vi "test_term2.vi"   [LabVIEW 2010]
uses:
  socket_type.ctl
  zmq_context.lvclass
  zmq_socket.lvclass
  zeromq.lvlib
types:
  T1 = typedef "zeromq.lvlib/socket_type.ctl" = enum8{"ZMQ_PAIR", "ZMQ_PUB", "ZMQ_SUB", "ZMQ_REQ", "ZMQ_REP", "ZMQ_DEALER", "ZMQ_ROUTER", "ZMQ_PULL", "ZMQ_PUSH", "ZMQ_XPUB", "ZMQ_XSUB"}
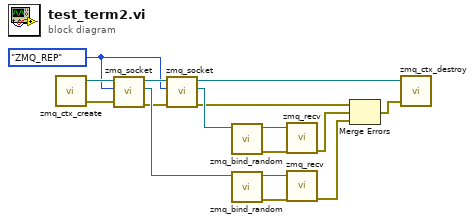
[diagram p0: block diagram]
diagram:
  w1 = socket_type."ZMQ_REP" ("socket type")
  n1 = call "zmq_ctx_create.vi"() -> ("error out"=w8:errorcluster, "context out"=w16:refnum<class "zmq_context.lvclass">)  [unwired: 4 in]
  n2 = call "zmq_socket.vi"("error in"=w8, "socket type"=w1, "context in"=w16) -> ("error out"=w7:errorcluster, "socket out"=w14:refnum<class "zmq_socket.lvclass">, "context out"=w15:refnum<class "zmq_context.lvclass">)  [unwired: 2 in]
  n3 = call "zmq_socket.vi"("error in"=w7, "socket type"=w1, "context in"=w15) -> ("error out"=w6:errorcluster, "socket out"=w13:refnum<class "zmq_socket.lvclass">, "context out"=w2:refnum<class "zmq_context.lvclass">)  [unwired: 2 in]
  n4 = call "zmq_bind_random.vi"("socket in"=w13) -> ("error out"=w12:errorcluster, "socket out"=w11:refnum<class "zmq_socket.lvclass">)  [unwired: 3 in, 2 out]
  n5 = call "zmq_bind_random.vi"("socket in"=w14) -> ("error out"=w9:errorcluster, "socket out"=w10:refnum<class "zmq_socket.lvclass">)  [unwired: 3 in, 2 out]
  n6 = call "zmq_recv.vi"("error in"=w12, "socket in"=w11) -> ("error out"=w5:errorcluster)  [unwired: 3 in, 4 out]
  n7 = call "zmq_recv.vi"("error in"=w9, "socket in"=w10) -> ("error out"=w4:errorcluster)  [unwired: 3 in, 4 out]
  n8 = Merge Errors(w6, w5, w4) -> (w3:errorcluster)
  n9 = call "zmq_ctx_destroy.vi"("error in"=w3, "context in"=w2) -> ()  [unwired: 3 in, 1 out]
